vi "testMyrioCounter.vi"() -> ()   [LabVIEW 2015]
uses:
  <vilib>/rvi/Emulation/niFpgaGetClockAttributes.vi
  <vilib>/rvi/Emulation/niFpgaSctlEmulationGetInTimedLoop.vi
  <vilib>/rvi/Emulation/niFpgaEmulationReportErrorSimple.vi
  <vilib>/rvi/eio/common/nirviEmuTemplateMethod_errors.vi
  <vilib>/rvi/Memory/Memory_Emulation/nirvimemoryEmulation.vi
  <vilib>/rvi/Memory/Memory_Emulation/nirvimemoryFastEmulation.vi
  <vilib>/rvi/DataTransferAndStorage/Container/Common/niFpgaContainerGetUniqueNameForEmu.vi
  <vilib>/rvi/Memory/Memory_Emulation/niFpgaMemoryEmulationCacheClearOnFirstRun.vi
  <vilib>/rvi/Memory/Memory_Emulation/nirvimemoryEmulationManagerCache_MakeExclusive.vi
  <vilib>/rvi/Memory/Memory_Emulation/niFpgaMemoryEmulationValidateCache.vi
  <vilib>/rvi/Memory/Memory_Emulation/nirvimemoryEmulationManagerCache_InsertValue.vi
  <vilib>/Utility/error.llb/Clear Errors.vi
  <vilib>/rvi/Memory/Memory_Emulation/nirvimemoryEmulationManagerCache_ReleaseExclusive.vi
  <vilib>/rvi/Memory/Memory_Emulation/nirvimemoryEmulationManagerCache_GetValue.vi
  <vilib>/rvi/Emulation/niFpgaEmulationIsFPGAContextNoSignature.vi
  <vilib>/rvi/Memory/Memory_Emulation/nirvimemoryEmulationManagerCache_SetValue.vi
  <vilib>/rvi/Emulation/niFpgaSctlEmulationResourceMgr.vi
  <vilib>/rvi/Emulation/niFpgaCriticalErrorInLSC.vi
  <vilib>/rvi/Emulation/niFpgaProcessEmulError.vi
  <vilib>/rvi/interface/RandomDataEmulation/niFpgaRandomDataHandleErrors.vi
  <vilib>/eio/EIONode/EIONode.xnode
  <vilib>/rvi/DataTransferAndStorage/Container/XNode/niFpgaContainer.xnode
  <vilib>/rvi/interface/RandomDataEmulation/nirviRandomDataFpgaReadWriteTemplate.vi
panel:
  in  "Trigperscan":u32=160
  out "Timed Out?":bool
  in  "FIFO_Timeout":i32=40000
  in  "VC_pt_in_fifo":i32=2048
  in  "YStpMPlsInFifo":i32
  in  "Sine":bool=TRUE
  in  "stop":bool
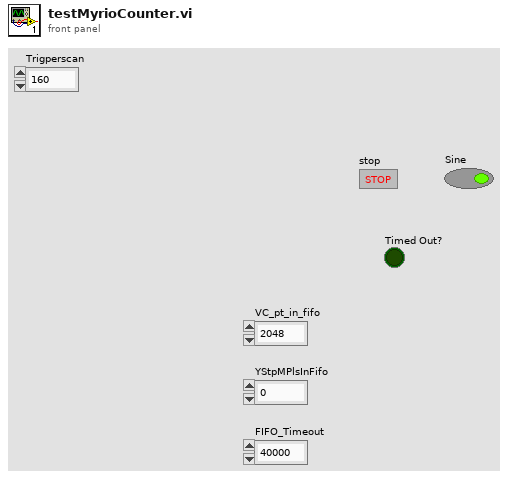
[diagram p1: front panel]
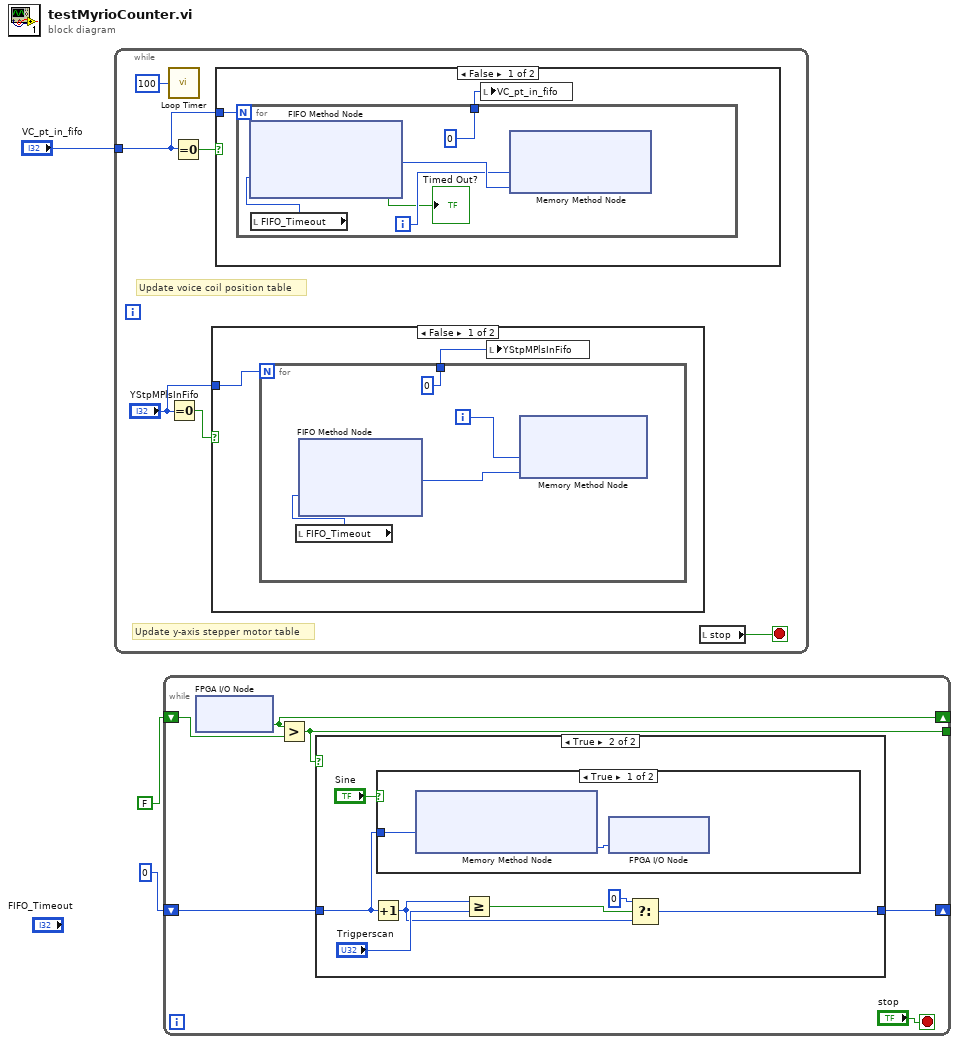
[diagram p0: block diagram]
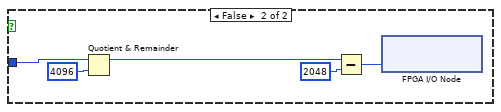
[diagram p3: hidden frame]
diagram:
  n1 = while {
    tunnel: "VC_pt_in_fifo" -> [w4]
    stop <- w5 stop-if-true
    # "Update y-axis stepper motor table"
    # "Update voice coil position table"
    n2 = call "Loop Timer"("Count(Ticks)"=u8 100) -> ()  [unwired: 1 out]
    n3 = Equal To 0?(x="YStpMPlsInFifo") -> (x = 0?=w7:bool)
    n4 = Equal To 0?(x=w4) -> (x = 0?=w9:bool)
    n5 = case shown="False" w7 {
      tunnel: "YStpMPlsInFifo" -> [w11 _]
      frame False {
        n6 = for {
          N: w11 -> [_]
          tunnel: [0] -> w10
          i -> [w13]
          n7 = local read "FIFO_Timeout"() -> (w15:i32)
          n8 = xnode ("FIFO Method Node")("Timeout"=w15) -> ("Element"=w14:u32)  [unwired: 1 in, 2 out]
          n9 = xnode ("Memory Method Node")("Address"=w13, "Data"=w14) -> ()  [unwired: 1 in, 1 out]
        }
        n10 = local write "YStpMPlsInFifo"(w10) -> ()
      }
      frame True {
      }
    }
    n11 = case shown="False" w9 {
      tunnel: w4 -> [w17 _]
      frame False {
        n12 = for {
          N: w17 -> [_]
          tunnel: [i16 0] -> w16
          i -> [w20]
          n13 = local read "FIFO_Timeout"() -> (w21:i32)
          n14 = xnode ("FIFO Method Node")("Timeout"=w21) -> ("Element"=w22:i16, "Timed Out?"=→"Timed Out?":bool)  [unwired: 1 in, 1 out]
          n15 = xnode ("Memory Method Node")("Address"=w20, "Data"=w22) -> ()  [unwired: 1 in, 1 out]
        }
        n16 = local write "VC_pt_in_fifo"(w16) -> ()
      }
      frame True {
      }
    }
    n17 = local read "stop"() -> (w5:bool)
  }
  n18 = while {
    shift-right: [w23] -> _
    shift-left: FALSE -> [w28]
    tunnel: [w27] -> _
    shift-right: [w25] -> _
    shift-left: u32 0 ("Numeric") -> [w26]
    stop <- "stop" stop-if-true
    n19 = xnode "FPGA I/O Node"() -> ("Trig in"=w23:bool)  [unwired: 1 in, 1 out]
    n20 = Greater?(x=w23, y=w28) -> (0:w27:bool)
    n21 = case shown="True" w27 {
      tunnel: w26 -> [w29 w30]
      tunnel: [w29 w31] -> w25
      frame False {
      }
      frame True {
        n22 = Increment(x=w30) -> (x+1=w32:u32)
        n23 = case shown="True" "Sine" {
          tunnel: w30 -> [w37 w43]
          frame True {
            n24 = xnode ("Memory Method Node")("Address"=w37) -> ("Data"=w38:i16)  [unwired: 1 in, 1 out]
            n25 = xnode "FPGA I/O Node"("Fast Mirror"=w38) -> ()  [unwired: 1 in, 1 out]
          }
          frame False {
            n26 = Quotient & Remainder(x=w43, y=4096) -> (x-y*floor(x/y)=w41:u32)  [unwired: 1 out]
            n27 = Subtract(x=w41, y=u32 2048) -> (x-y=w39:u32)
            n28 = xnode "FPGA I/O Node"("Fast Mirror"=w39) -> ()  [unwired: 1 in, 1 out]
          }
        }
        n29 = Greater Or Equal?(x=w32, y="Trigperscan") -> (x >= y?=w34:bool)
        n30 = Select(t=u32 0, s=w34, f=w32) -> (s? t:f=w31:u32)
      }
    }
  }
